vi "DestroyAll.vi"(8 "error in (no error)":errorcluster) -> (0 "error out":errorcluster)   [LabVIEW 2021, in "Application.lvclass"]
uses:
  Application.lvclass
  Interface_Object_ICreateDestroy/ICreateDestroy/ICreateDestroy.lvclass
  f84cd1a8-cfe3-4f9a-8f5c-77164aa315c0.vi
  <vilib>/TriekselSoft/TracerLibrary/TracerLibrary/Tracer/protected/SendMessage.vi
  <vilib>/TriekselSoft/TracerLibrary/TracerLibrary/Tracer/protected/Timestamp.vi
  <vilib>/TriekselSoft/TracerLibrary/TracerLibrary/Tracer/Tracer_Level-Debug.vi
  <vilib>/TriekselSoft/TracerLibrary/TracerLibrary/Tracer/protected/Tracer_ClassAttributes.vi
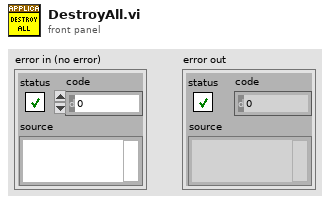
[diagram p1: front panel]
types:
  T1 = typedef "Application.lvclass/ObjectAttributes.ctl" = cluster{"Objects":variant, "BasePath":path, "Application":refnum<class "Application.lvclass">}
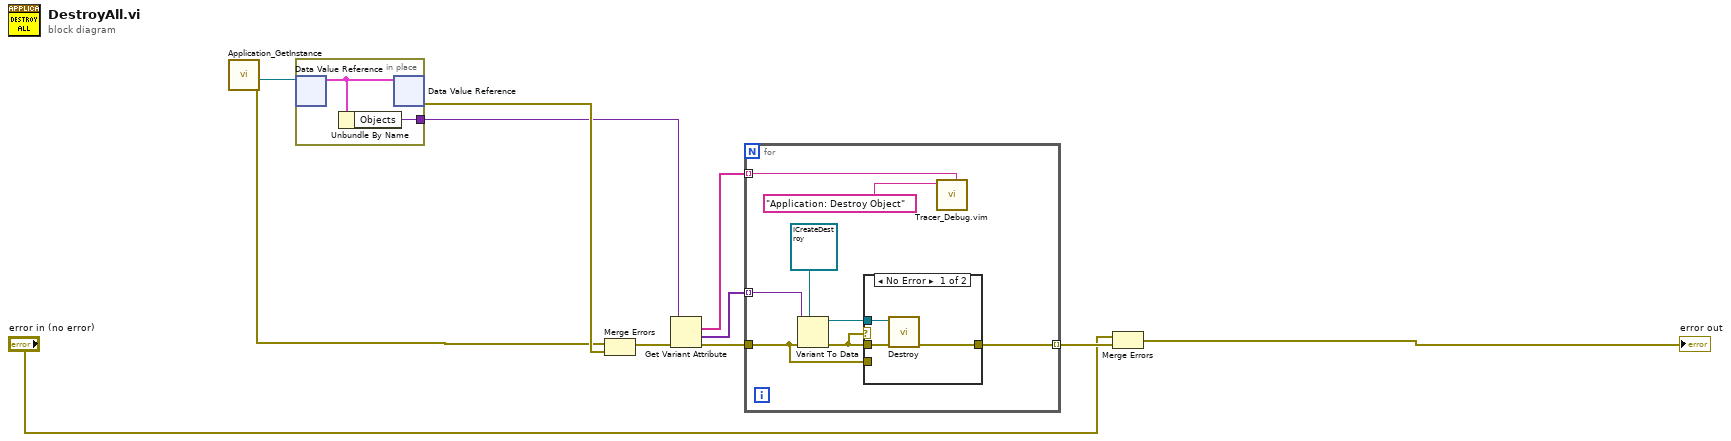
[diagram p0: block diagram]
diagram:
  n1 = call "Application_GetInstance.vi"() -> ("error out"=w6:errorcluster, "DVRRefOut"=w9:refnum<data-value>)  [unwired: 7 in, 3 out]
  n2 = in-place {
    in-place-border: [w12] -> w7
    n3 = in-place-dvr #1(w9) -> (w13:T1)  [unwired: 1 out]
    n4 = Unbundle By Name(w13) -> ("Objects"=w12:variant)
    n5 = in-place-dvr #1(w13) -> (w10:errorcluster)  [unwired: 1 out]
  }
  n6 = Merge Errors(w6, w10) -> (w8:errorcluster)
  n7 = Get Variant Attribute(Variant=w7, error in=w8) -> (names=w1:string[], values=w4:variant[], error out=w5:errorcluster)  [unwired: 2 in, 1 out]
  n8 = for {
    tunnel: w5 -> [w16]
    tunnel: w4 -> [w21] mode=indexing
    tunnel: [w18] -> w3 mode=indexing
    tunnel: w1 -> [w14] mode=indexing
    n9 = Variant To Data(error in=w16, type=refnum<class "ICreateDestroy.lvclass"> refnum ("ICreateDestroy"), Variant=w21) -> (data=w19:refnum<class "ICreateDestroy.lvclass">, error out=w17:errorcluster)
    n10 = case shown="No Error" w17 {
      tunnel: w17 -> [w24 _]
      tunnel: w19 -> [w23 _]
      tunnel: [w22 w25] -> w18
      tunnel: w16 -> [_ w25]
      frame No Error {
        n11 = call-dynamic "Destroy.vi"("Error In"=w24, "object in"=w23) -> ("Error Out"=w22:errorcluster)  [unwired: 8 in, 1 out]
      }
      frame Error {
      }
    }
    n12 = call "Tracer_Debug.vim"("Data"=w14, "Text"="Application: Destroy Object") -> ()  [unwired: 9 in, 1 out]
  }
  n13 = Merge Errors("error in (no error)", w3) -> (→"error out":errorcluster)
